vi "test.vi"(8 "error in (no error)":errorcluster, 11 "Cell in":refnum<class "Cell.lvclass">) -> (0 "error out":errorcluster, 3 "Boolean":bool)   [LabVIEW 2014, in "Cell.lvclass"]
uses:
  Cell.lvclass
  Cell.lvclass/Cell.ctl
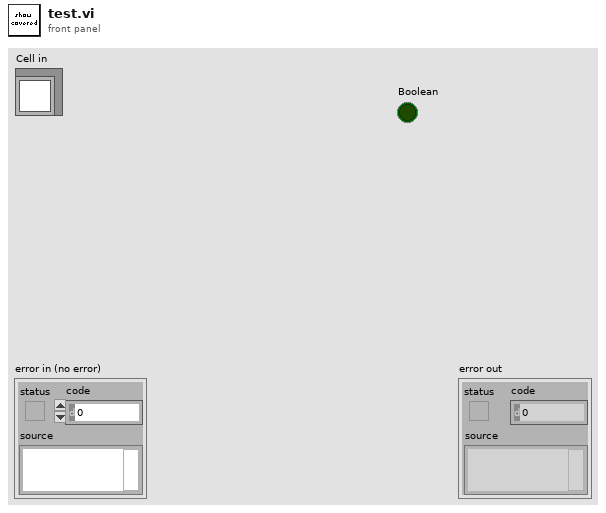
[diagram p1: front panel]
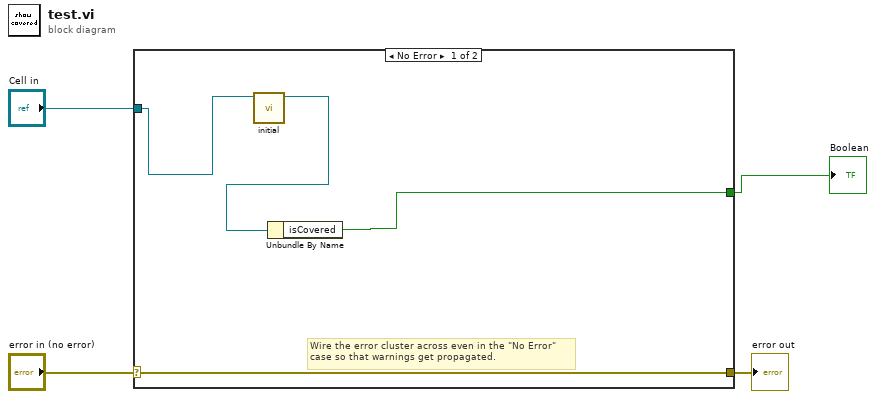
[diagram p0: block diagram]
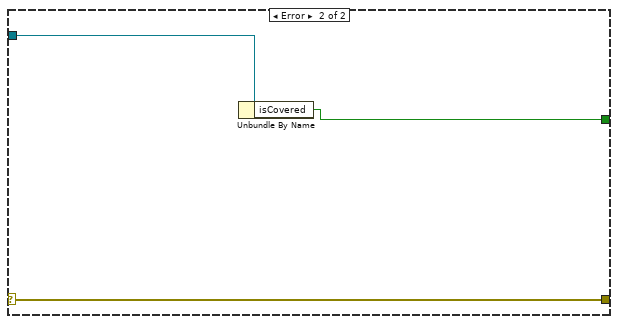
[diagram p2: hidden frame]
diagram:
  n1 = case shown="No Error" "error in (no error)" {
    selector: "error in (no error)" -> [w8 w11]
    tunnel: [w8 w11] -> w3
    tunnel: "Cell in" -> [w6 w10]
    tunnel: [w7 w9] -> w1
    frame No Error {
      # "Wire the error cluster across even in the \"No Error\"\ncase so that warnings get propagated."
      n2 = call-dynamic "initial.vi"("Cell in"=w6) -> ("Cell out"=w5:refnum<class "Cell.lvclass">)  [unwired: 9 in, 1 out]
      n3 = Unbundle By Name(w5) -> ("isCovered"=w7:bool)
    }
    frame Error {
      n4 = Unbundle By Name(w10) -> ("isCovered"=w9:bool)
    }
  }
  "error out" <- w3
  "Boolean" <- w1
